vi "emi_Reinit all controls to default.vi"(5 "VI Refnum(This vi)":refnum<vi>, 9 "error in (no error)":errorcluster) -> (6 "VI Refnum":refnum<vi>, 10 "error out":errorcluster)   [LabVIEW 2011]
doc: "Reinitialise all controls on VI to default values. \n\nIf no VI ref in, then the VI containing this VI is used.\n\nOn error in: Does not run."
panel:
  # "Set all controls to default"
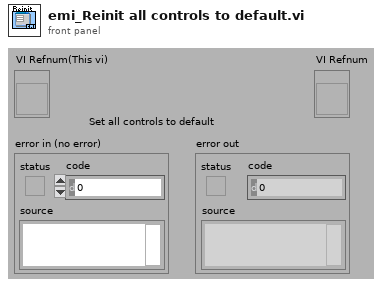
[diagram p1: front panel]
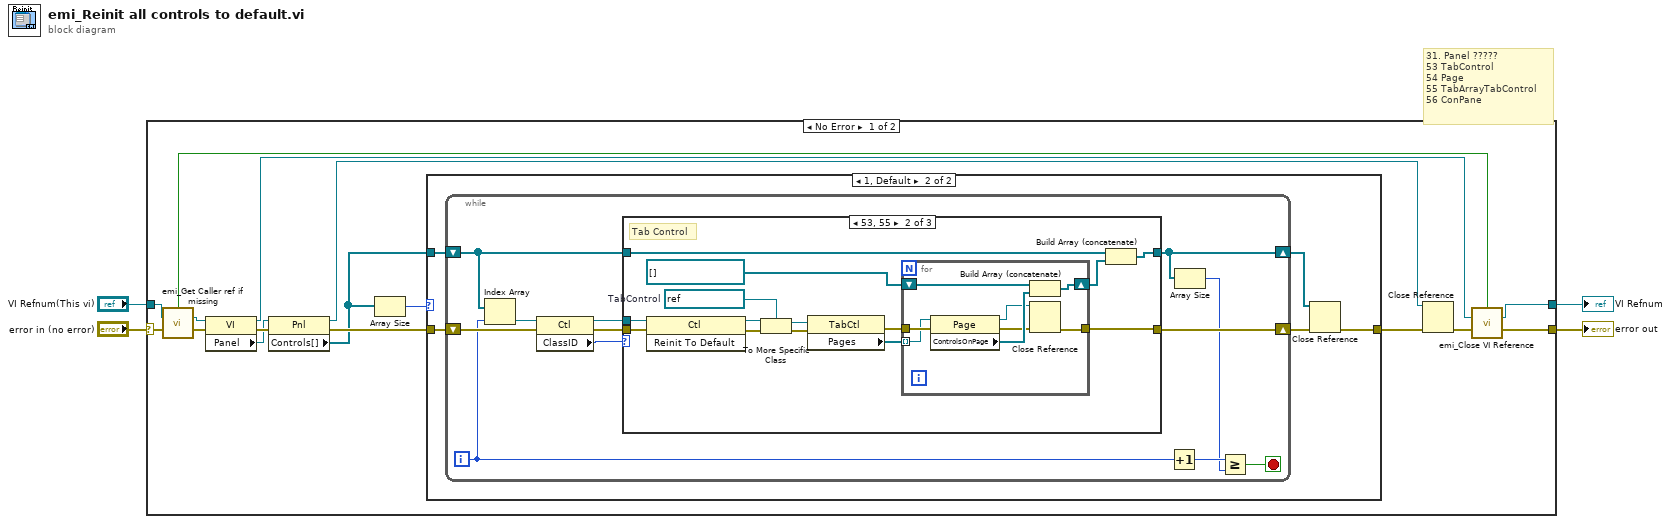
[diagram p0: block diagram]
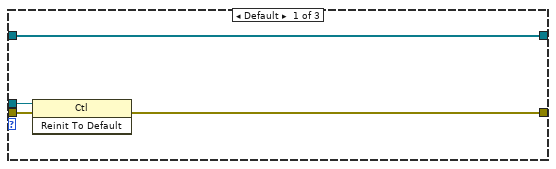
[diagram p3: hidden frame]
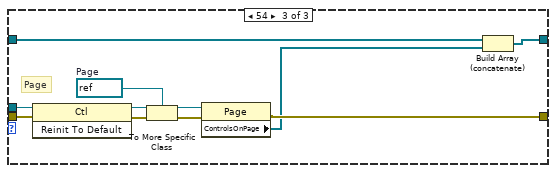
[diagram p4: hidden frame]
diagram:
  # "31. Panel ?????\n53 TabControl \n54 Page \n55 TabArrayTabControl \n56 ConPane"
  n1 = case shown="No Error" "error in (no error)" {
    selector: "error in (no error)" -> [w12 w77]
    tunnel: [w14 w77] -> w4
    tunnel: "VI Refnum(This vi)" -> [w10 w76]
    tunnel: [w13 w76] -> w2
    frame No Error {
      n2 = call "emi_Get Caller ref if missing.vi"("VI Refnum(Calling VI)"=w10, "error in (no error)"=w12) -> ("Ref Generated"=w17:bool, "VI Refnum Out"=w9:refnum<vi>, "error out"=w11:errorcluster)  [unwired: 11 in]
      n3 = property class="VI"(reference=w9, error in=w11) -> (reference out=w8:refnum<vi>, error out=w20:errorcluster, "Panel"=w16:refnum<vi>)
      n4 = property class="Pnl"(reference=w16, error in=w20) -> (reference out=w18:refnum<vi>, error out=w19:errorcluster, "Controls[]"=w6:refnum<vi>[])
      n5 = Array Size(array=w6) -> (size(s)=w5:i32)
      n6 = case shown="1, Default" w5 {
        tunnel: w19 -> [w21 w26]
        tunnel: w6 -> [_ w24]
        tunnel: [w21 w23] -> w7
        frame 0 {
        }
        frame 1, Default {
          n7 = while {
            shift-right: [w38] -> w25
            shift-left: w26 -> [w35]
            shift-right: [w31] -> w22
            shift-left: w24 -> [w33]
            i -> [w30]
            stop <- w27 stop-if-true
            n8 = Index Array(array=w33, index=w30) -> (element=w32:refnum<vi>)
            n9 = property class="Ctl"(reference=w32, error in=w35) -> (reference out=w37:refnum<vi>, error out=w36:errorcluster, "ClassID"=w34:u32)
            n10 = case shown="53, 55" w34 {
              tunnel: [w39 w46 w66] -> w38
              tunnel: w37 -> [w42 w56 w75]
              tunnel: w36 -> [w41 w55 w74]
              tunnel: w33 -> [w40 w49 w68]
              tunnel: [w40 w48 w67] -> w31
              frame Default {
                n11 = invoke class="Ctl" method="Reinit To Default"(reference=w42, error in=w41) -> (error out=w39:errorcluster)  [unwired: 1 in, 2 out]
              }
              frame 53, 55 {
                w50 = refnum<vi> refnum  # TabControl
                # "Tab Control"
                n12 = invoke class="Ctl" method="Reinit To Default"(reference=w56, error in=w55) -> (reference out=w52:refnum<vi>, error out=w53:errorcluster)  [unwired: 1 in, 1 out]
                n13 = To More Specific Class(target class=w50, reference=w52, error in=w53) -> (specific class reference=w51:refnum<vi>, error out=w54:errorcluster)
                n14 = property class="TabCtl"(reference=w51, error in=w54) -> (error out=w47:errorcluster, "Pages"=w45:refnum<vi>[])  [unwired: 1 out]
                n15 = for {
                  tunnel: w47 -> [w64]
                  tunnel: [w58] -> w46
                  tunnel: w45 -> [w63] mode=indexing
                  shift-right: [w60] -> w43
                  shift-left: refnum<vi>[] [] ("Controls on Page[]") -> [w62]
                  n16 = property class="Page"(reference=w63, error in=w64) -> (reference out=w57:refnum<vi>, error out=w59:errorcluster, "ControlsOnPage"=w61:refnum<vi>[])
                  n17 = Build Array (concatenate)(w62, w61) -> (w60:refnum<vi>[])
                  n18 = Close Reference(reference=w57, error in (no error)=w59) -> (error out=w58:errorcluster)
                }
                n19 = Build Array (concatenate)(w49, w43) -> (w48:refnum<vi>[])
              }
              frame 54 {
                w71 = refnum<vi> refnum  # Page
                # "Page"
                n20 = invoke class="Ctl" method="Reinit To Default"(reference=w75, error in=w74) -> (reference out=w72:refnum<vi>, error out=w73:errorcluster)  [unwired: 1 in, 1 out]
                n21 = To More Specific Class(target class=w71, reference=w72, error in=w73) -> (specific class reference=w69:refnum<vi>, error out=w70:errorcluster)
                n22 = property class="Page"(reference=w69, error in=w70) -> (error out=w66:errorcluster, "ControlsOnPage"=w65:refnum<vi>[])  [unwired: 1 out]
                n23 = Build Array (concatenate)(w68, w65) -> (w67:refnum<vi>[])
              }
            }
            n24 = Increment(x=w30) -> (x+1=w29:i32)
            n25 = Array Size(array=w31) -> (size(s)=w28:i32)
            n26 = Greater Or Equal?(x=w29, y=w28) -> (x >= y?=w27:bool)
          }
          n27 = Close Reference(reference=w22, error in (no error)=w25) -> (error out=w23:errorcluster)
        }
      }
      n28 = Close Reference(reference=w18, error in (no error)=w7) -> (error out=w15:errorcluster)
      n29 = call "emi_Close VI Reference.vi"("Close ref?(T)"=w17, "VI Refnum"=w8, "error in (no error)"=w15) -> ("VI Refnum Out"=w13:refnum<vi>, "error out"=w14:errorcluster)  [unwired: 11 in]
    }
    frame Error {
    }
  }
  "error out" <- w4
  "VI Refnum" <- w2
